vi "ArrayDimensions.vi"() -> ()   [LabVIEW 2019]
panel:
  out "4DArray 2":dbl[][][][](array[numeric])
  out "3DArray 2":dbl[][][](array[numeric])
  out "2DArray 2":dbl[][](array[numeric])
  out "1DArray 2":dbl[](array[numeric])
  out "Numeric 2":dbl
  in  "4DArray":dbl[][][][](array[numeric])
  in  "3DArray":dbl[][][](array[numeric])
  in  "2DArray":dbl[][](array[numeric])
  in  "Numeric":dbl
  in  "1DArray":dbl[](array[numeric])
  # "1"
  # "1"
  # "2"
  # "1"
  # "2"
  # "3"
  # "1"
  # "2"
  # "3"
  # "4"
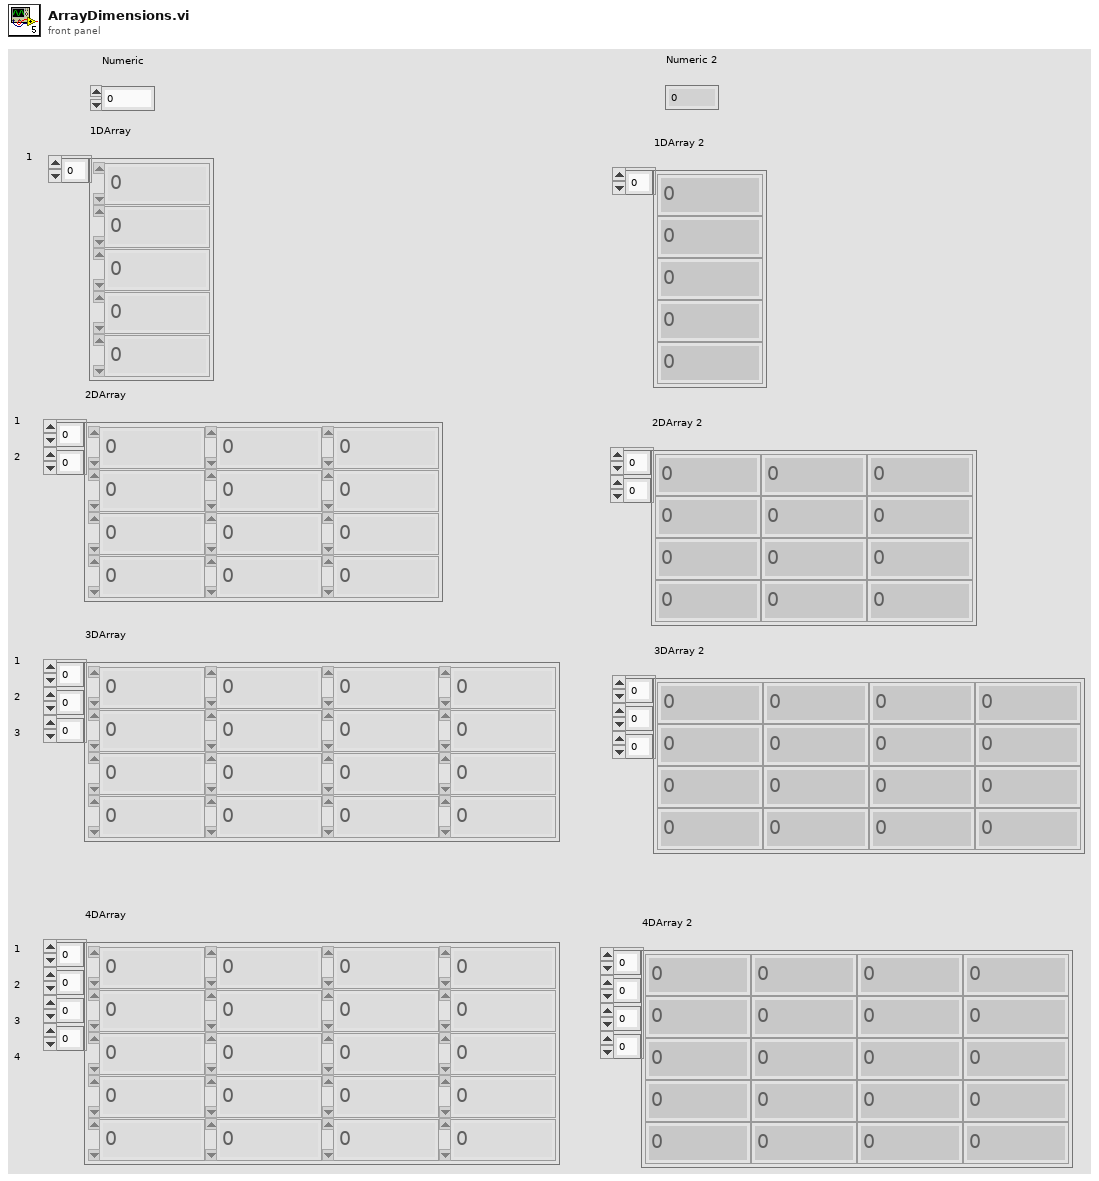
[diagram p1: front panel]
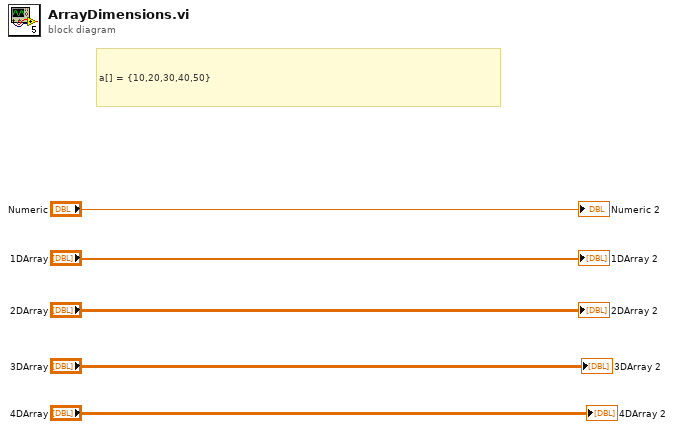
[diagram p0: block diagram]
diagram:
  # "a[] = {10,20,30,40,50}"
  "Numeric 2" <- "Numeric"
  "1DArray 2" <- "1DArray"
  "2DArray 2" <- "2DArray"
  "3DArray 2" <- "3DArray"
  "4DArray 2" <- "4DArray"
